vi "XML_ControlConfig.vi"(8 "error in (no error)":errorcluster, 9 "Save?(T)":bool=TRUE) -> (0 "error out":errorcluster)   [LabVIEW 2012]
uses:
  <vilib>/Utility/xml.llb/Read From XML File(array).vi
  <vilib>/Utility/xml.llb/Write to XML File(array).vi
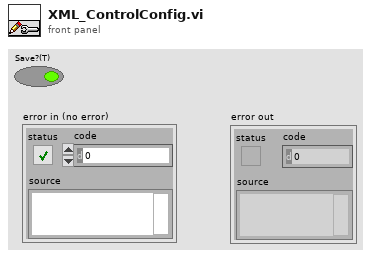
[diagram p1: front panel]
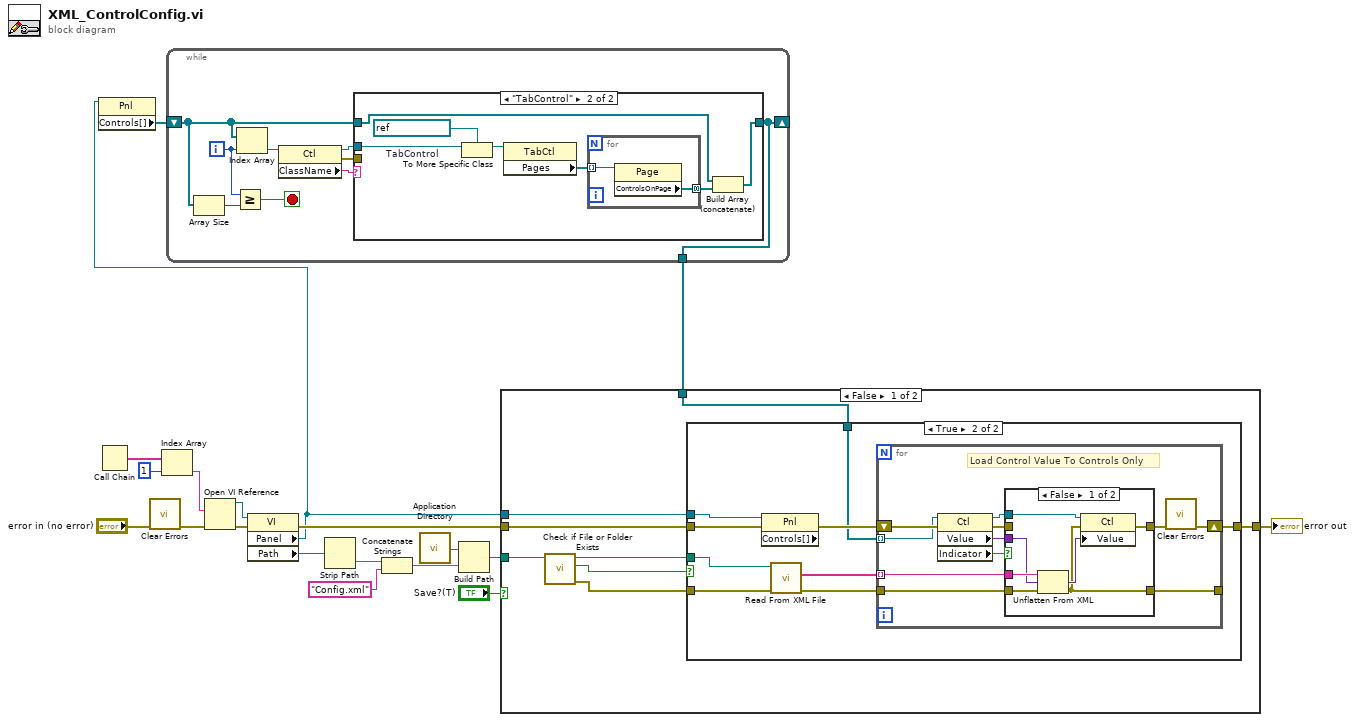
[diagram p0: block diagram]
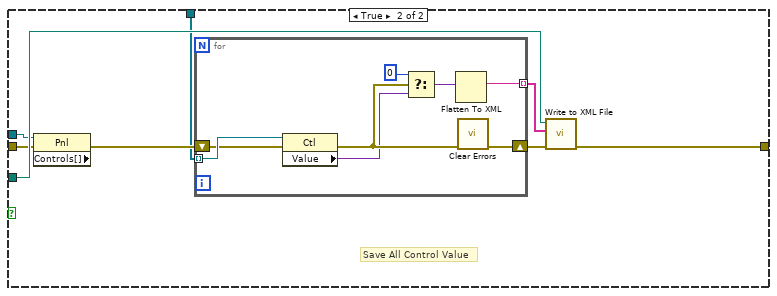
[diagram p5: hidden frame]
diagram:
  n1 = Call Chain() -> (call chain=w16:string[])
  n2 = call <vilib>:"Clear Errors.vi"("error in (no error)"="error in (no error)") -> ("error out"=w4:errorcluster)  [unwired: 6 in]
  n3 = Index Array(array=w16, index=1) -> (element=w14:string)
  n4 = Open VI Reference(vi path=w14, error in (no error)=w4) -> (vi reference=w13:refnum<vi>, error out=w7:errorcluster)  [unwired: 4 in]
  n5 = property class="VI"(reference=w13, error in=w7) -> (error out=w17:errorcluster, "Panel"=w2:refnum<vi>, "Path"=w12:path)  [unwired: 1 out]
  n6 = property class="Pnl"(reference=w2) -> ("Controls[]"=w3:refnum<vi>[])  [unwired: 1 in, 2 out]
  n7 = while {
    shift-right: [w20] -> _
    shift-left: w3 -> [w25]
    tunnel: [w20] -> w1
    i -> [w24]
    stop <- w22 stop-if-true
    n8 = Array Size(array=w25) -> (size(s)=w23:i32)
    n9 = Greater Or Equal?(x=w24, y=w23) -> (x >= y?=w22:bool)
    n10 = Index Array(array=w25, index=w24) -> (element=w26:refnum<vi>)
    n11 = property class="Ctl"(reference=w26) -> (reference out=w27:refnum<vi>, error out=w21:errorcluster, "ClassName"=w28:string)  [unwired: 1 in]
    n12 = case shown="\"TabControl\"" w28 {
      tunnel: w27 -> [_ w35]
      tunnel: [w29 w31] -> w20
      tunnel: w25 -> [w29 w32]
      tunnel: w21 -> [_ _]
      frame Default {
      }
      frame "TabControl" {
        w34 = refnum<vi> refnum  # TabControl
        n13 = To More Specific Class(target class=w34, reference=w35) -> (specific class reference=w36:refnum<vi>)  [unwired: 1 in, 1 out]
        n14 = property class="TabCtl"(reference=w36) -> ("Pages"=w33:refnum<vi>[])  [unwired: 1 in, 2 out]
        n15 = for {
          tunnel: w33 -> [w38] mode=indexing
          tunnel: [w37] -> w30 mode=concatenating
          n16 = property class="Page"(reference=w38) -> ("ControlsOnPage"=w37:refnum<vi>[])  [unwired: 1 in, 2 out]
        }
        n17 = Build Array (concatenate)(w32, w30) -> (w31:refnum<vi>[])
      }
    }
  }
  n18 = Strip Path(path=w12) -> (name=w10:string)  [unwired: 1 out]
  n19 = Concatenate Strings(w10, "Config.xml" ("string")) -> (w9:string)
  n20 = call <vilib>:"Application Directory.vi"() -> ("Application Directory"=w11:path)
  n21 = Build Path(base path=w11, name or relative path=w9) -> (appended path=w19:path)
  n22 = case shown="False" "Save?(T)" {
    tunnel: w19 -> [w46 w81]
    tunnel: [w42 w78] -> w18
    tunnel: w17 -> [w40 w79]
    tunnel: w2 -> [w41 w80]
    tunnel: w1 -> [w39 w77]
    frame False {
      n23 = call <vilib>:"Check if File or Folder Exists.vi"("path"=w46) -> ("error out"=w43:errorcluster, "file or folder exists?"=w45:bool, "dup path"=w44:path)  [unwired: 8 in]
      n24 = case shown="True" w45 {
        tunnel: w44 -> [_ w56]
        tunnel: w43 -> [_ w55]
        tunnel: [w47 w52] -> w42
        tunnel: w41 -> [_ w53]
        tunnel: w40 -> [w47 w50]
        tunnel: w39 -> [_ w48]
        frame False {
        }
        frame True {
          n25 = property class="Pnl" props=["Controls[]"](reference=w53, error in=w50) -> (error out=w54:errorcluster)  [unwired: 2 out]
          n26 = call-poly <vilib>:"Read From XML File.vi"("error in (no error)"=w55, "XML File Path"=w56) -> ("error out"=w49:errorcluster, "XML Elements"=w51:string[])  [unwired: 7 in, 1 out]
          n27 = for {
            tunnel: w48 -> [w62] mode=indexing
            shift-right: [w66] -> w52
            shift-left: w54 -> [w63]
            tunnel: w51 -> [w65] mode=indexing
            tunnel: w49 -> [w59]
            tunnel: [w58] -> _
            # "Load Control Value To Controls Only"
            n28 = property class="Ctl"(reference=w62, error in=w63) -> (reference out=w61:refnum<vi>, error out=w60:errorcluster, "Value"=w64:variant, "Indicator"=w57:bool)
            n29 = case shown="False" w57 {
              tunnel: [w74 w76] -> w67
              tunnel: w65 -> [w73 _]
              tunnel: w64 -> [w71 _]
              tunnel: w61 -> [w70 _]
              tunnel: w60 -> [_ w76]
              tunnel: w59 -> [w69 w75]
              tunnel: [w68 w75] -> w58
              frame False {
                n30 = Unflatten From XML(xml string=w73, type=w71, error in (no error)=w69) -> (value=w72:variant, error out=w68:errorcluster)
                n31 = property class="Ctl"(reference=w70, error in=w68, "Value"=w72) -> (error out=w74:errorcluster)  [unwired: 1 out]
              }
              frame True {
                # "ignore indicator"
              }
            }
            n32 = call <vilib>:"Clear Errors.vi"("error in (no error)"=w67) -> ("error out"=w66:errorcluster)  [unwired: 6 in]
          }
        }
      }
    }
    frame True {
      # "Save All Control Value"
      n33 = property class="Pnl" props=["Controls[]"](reference=w80, error in=w79) -> (error out=w82:errorcluster)  [unwired: 2 out]
      n34 = for {
        tunnel: w77 -> [w92] mode=indexing
        shift-right: [w90] -> w83
        shift-left: w82 -> [w91]
        tunnel: [w85] -> w84 mode=indexing
        n35 = property class="Ctl"(reference=w92, error in=w91) -> (error out=w89:errorcluster, "Value"=w87:variant)  [unwired: 1 out]
        n36 = Select(t=0, s=w89, f=w87) -> (s? t:f=w86:variant)
        n37 = Flatten To XML(anything=w86) -> (xml string=w85:string)
        n38 = call <vilib>:"Clear Errors.vi"("error in (no error)"=w89) -> ("error out"=w90:errorcluster)  [unwired: 6 in]
      }
      n39 = call-poly <vilib>:"Write to XML File.vi"("error in (no error)"=w83, "XML Input"=w84, "XML File Path"=w81) -> ("error out"=w78:errorcluster)  [unwired: 6 in, 2 out]
    }
  }
  "error out" <- w18
